vi "ballrackrange.vi"   [LabVIEW 2016, in "Test2.lvrbt"]
uses:
  Test2.lvrbt
  <vilib>/NXT/Block Support/NXT_InputPort.ctl
  <vilib>/NXT/Hardware/Plugins/Tetrix DC Motor/TetrixDCMotorAddress.ctl
  <vilib>/NXT/NXTIO Xnodes/NXTIONodeSubVIs/TETRIX IO Move DC Motors.vi
  <vilib>/NXT/Dual Mode Library/Waits/Wait_EV3_Ultrasonic_Centimeter_Closer.vi
  <vilib>/NXT/NXTIO Xnodes/NXTIONodeSubVIs/TETRIX IO Stop DC Motors.vi
  <vilib>/NXT/Dual Mode Library/Waits/Wait_Num.vi
  <vilib>/NXT/Dual Mode Library/Waits/Wait_Touch.vi
  <vilib>/NXT/Dual Mode Library/Waits/Wait_EV3_Ultrasonic_Centimeters_Further.vi
  <vilib>/NXT/Subs/LVHSConnector.ctl
  <vilib>/NXT/NXTIO Xnodes/AddressXNode/NXTIOAddress.xnode
  <vilib>/NXT/NXTIO Xnodes/NXTIOXNode/NXTIO.xnode
  <vilib>/NXT/LegoClasses/BrickReference/BrickReference.lvclass
types:
  T1 = typedef "NXT_InputPort.ctl" = u32
  T2 = typedef "TetrixDCMotorAddress.ctl" = i32
  T3 = typedef "LVHSConnector.ctl" = refnum<class "BrickReference.lvclass">
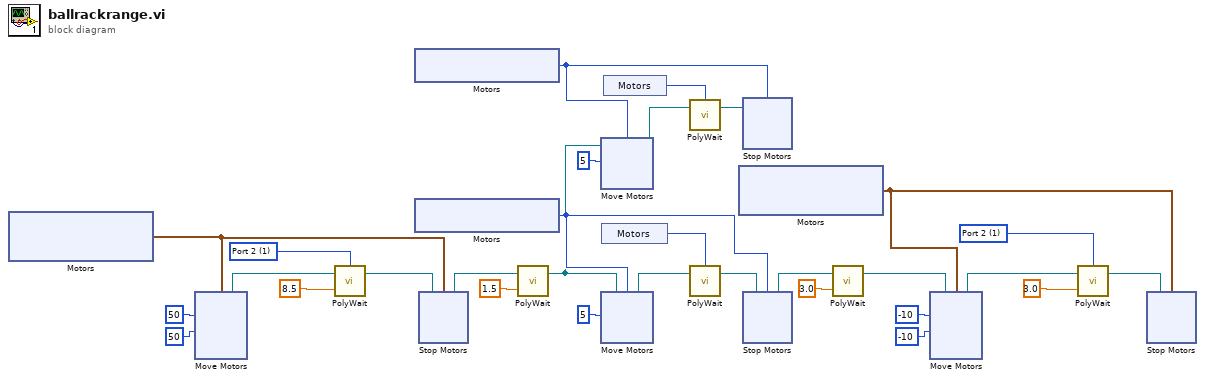
[diagram p0: block diagram]
diagram:
  w4 = T1 1 items=["Port 1", "Port 2", "Port 3", "Port 4"] ("Port (Port 1)")
  w11 = T1 1 items=["Port 1", "Port 2", "Port 3", "Port 4"] ("Port (Port 1)")
  n1 = xnode "Motors"() -> ("Motor"=w25:cluster{"TetrixDCMotor":T2, "TetrixDCMotor":T2})
  n2 = xnode "Move Motors"("Power/Speed 2"=i8 50, "Power/Speed 1"=i8 50, "Motors"=w25) -> ("NXT/EV3"=w28:T3)  [unwired: 1 in]
  n3 = call-poly <vilib>:"PolyWait.vi"("Centimeters (40)"=sgl 8.5, "NXT/EV3"=w28, "Port (Port 1)"=w11) -> ("NXT/EV3"=w26:T3)  [unwired: 1 in]
  n4 = xnode "Motors"() -> ("Motor"=w21:T2)
  n5 = xnode "Motors"() -> ("Motor"=w16:T2)
  n6 = xnode "Stop Motors"("Motors"=w25, "NXT/EV3"=w26) -> ("NXT/EV3"=w19:T3)
  n7 = call-poly <vilib>:"PolyWait.vi"("Time (1 sec)"=sgl 1.5, "NXT/EV3"=w19) -> ("NXT/EV3"=w14:T3)  [unwired: 2 in]
  n8 = xnode "Move Motors"("Power/Speed 1"=i8 5, "Motors"=w21, "NXT/EV3"=w14) -> ("NXT/EV3"=w23:T3)
  n9 = xnode "Move Motors"("Power/Speed 1"=i8 5, "Motors"=w16, "NXT/EV3"=w14) -> ("NXT/EV3"=w17:T3)
  n10 = xnode "Motors"() -> ("Sensor"=w13:T1)
  n11 = xnode "Motors"() -> ("Sensor"=w12:T1)
  n12 = call-poly <vilib>:"PolyWait.vi"("NXT/EV3"=w23, "Port (Port 1)"=w12) -> ("NXT/EV3"=w22:T3)  [unwired: 2 in]
  n13 = call-poly <vilib>:"PolyWait.vi"("NXT/EV3"=w17, "Port (Port 1)"=w13) -> ("NXT/EV3"=w15:T3)  [unwired: 2 in]
  n14 = xnode "Motors"() -> ("Motor"=w6:cluster{"TetrixDCMotor":T2, "TetrixDCMotor":T2})
  n15 = xnode "Stop Motors"("Motors"=w21, "NXT/EV3"=w22) -> ()  [unwired: 1 out]
  n16 = xnode "Stop Motors"("Motors"=w16, "NXT/EV3"=w15) -> ("NXT/EV3"=w10:T3)
  n17 = call-poly <vilib>:"PolyWait.vi"("Time (1 sec)"=sgl 3.0, "NXT/EV3"=w10) -> ("NXT/EV3"=w2:T3)  [unwired: 2 in]
  n18 = xnode "Move Motors"("Power/Speed 2"=i8 -10, "Power/Speed 1"=i8 -10, "Motors"=w6, "NXT/EV3"=w2) -> ("NXT/EV3"=w8:T3)
  n19 = call-poly <vilib>:"PolyWait.vi"("Centimeters (50)"=sgl 3.0, "NXT/EV3"=w8, "Port (Port 1)"=w4) -> ("NXT/EV3"=w7:T3)  [unwired: 1 in]
  n20 = xnode "Stop Motors"("Motors"=w6, "NXT/EV3"=w7) -> ()  [unwired: 1 out]
